vi "pitchVI.vi"() -> ()   [LabVIEW 2017]
uses:
  <vilib>/sound2/lvsound2.llb/Sound Output Task ID.ctl
  <vilib>/sound2/lvsound2.llb/Sound Output Write (DBL).vi
  <vilib>/sound2/lvsound2.llb/Sound File Write Open.vi
  <vilib>/sound2/lvsound2.llb/Sound File Write (DBL).vi
panel:
  in  "Clear":bool
  out "Sample Rate":dbl=48000.0
  in  "save":bool
  out "task ID out":T1=4294967295 format="%.0x"
  in  "Stop Play":bool
  in  "Pitch Shift \n(Octave)":i8
  in  "Shift":bool
  out "Right Channel":waveform(dbl)(graph)={"t0"=timestamp(0 s since 1904-01-01), "dt"=0.0020833333333333333, "Y"=[]}
  out "Left Channel":waveform(dbl)(graph)={"t0"=timestamp(0 s since 1904-01-01), "dt"=0.0020833333333333333, "Y"=[]}
  in  "waveform":dbl[][](array[numeric])
  in  "Stretch":bool
  in  "stop":bool
  in  "Play Signal":bool
  in  "Stretch Ratio":dbl=1.0
  in  "File to load":path
  # "Loneman's Phase Vocoder\nCopyright Jun D. Ouyang 06-06-2017"
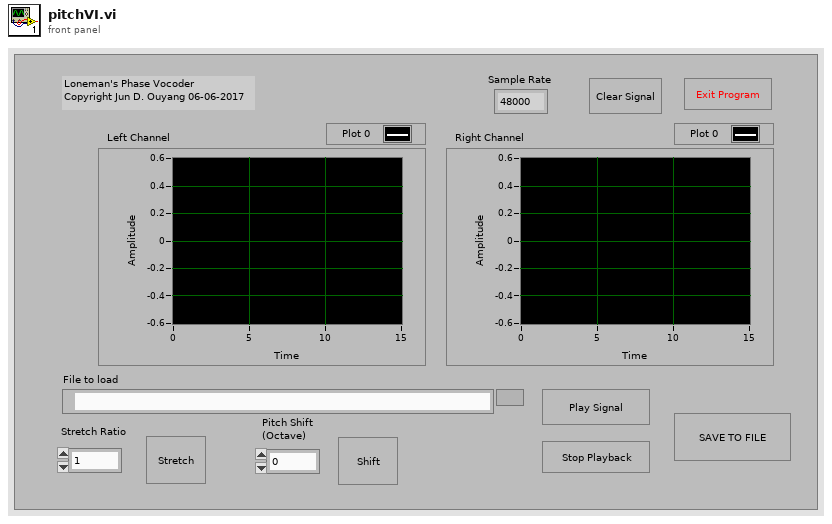
[diagram p1: front panel]
types:
  T1 = typedef "Sound Output Task ID.ctl" = u32
  T2 = typedef "Sound File Refnum.ctl" = refnum<file>
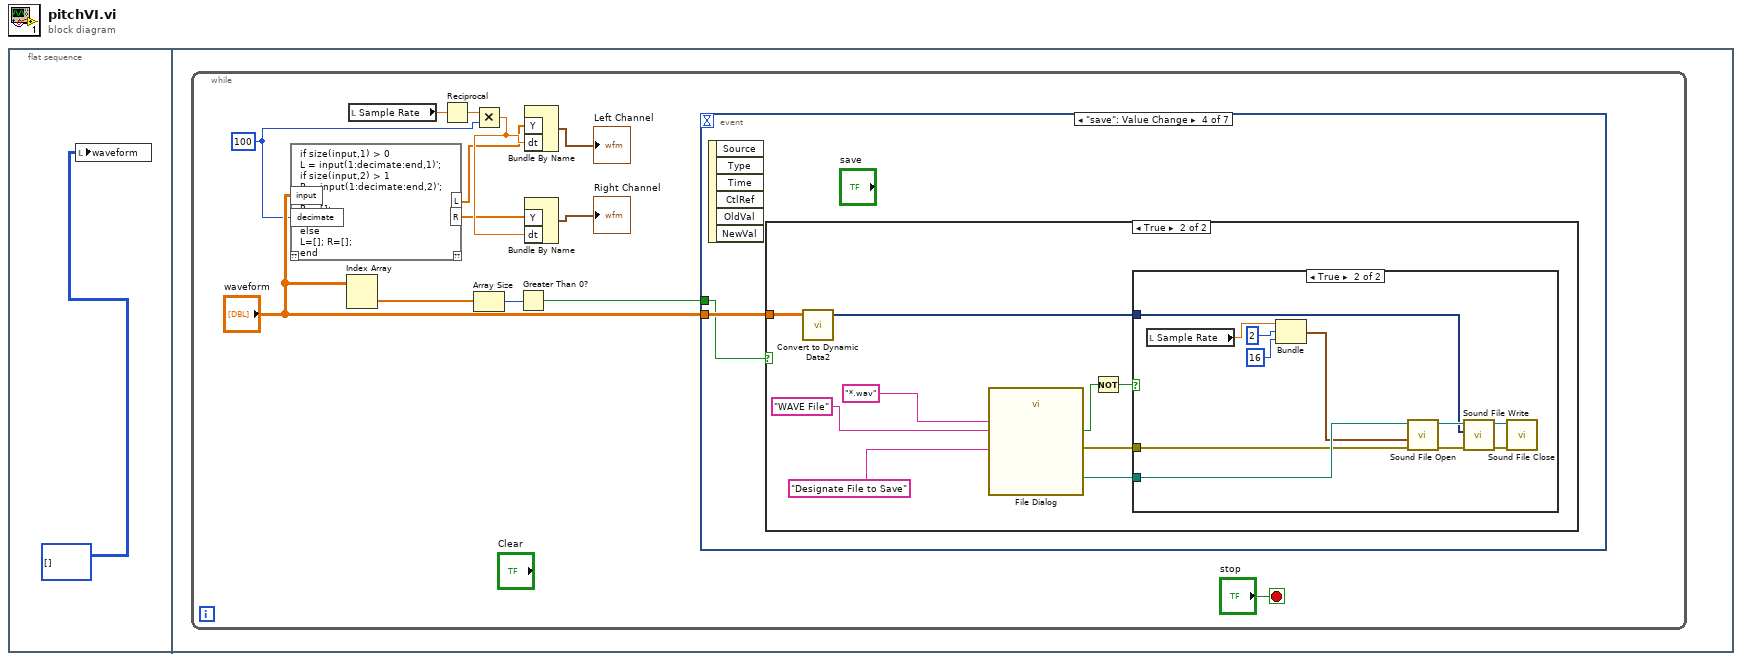
[diagram p0: block diagram]
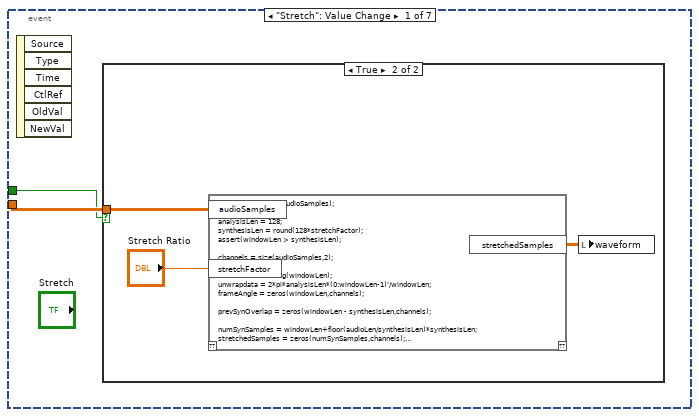
[diagram p2: hidden frame]
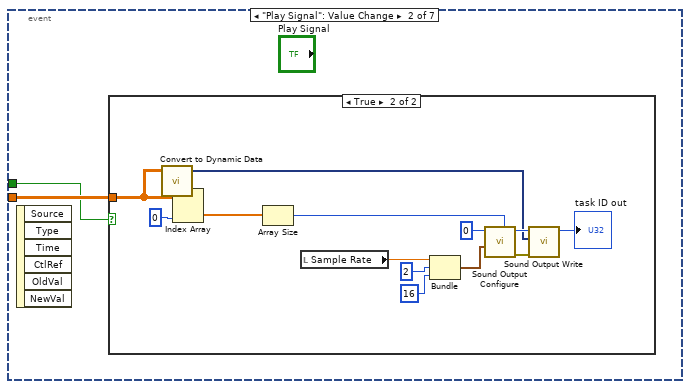
[diagram p4: hidden frame]
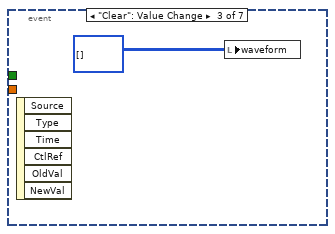
[diagram p6: hidden frame]
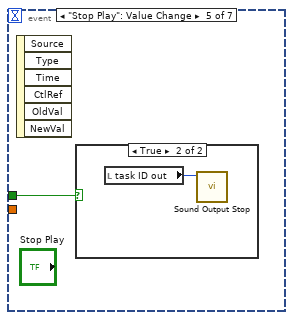
[diagram p9: hidden frame]
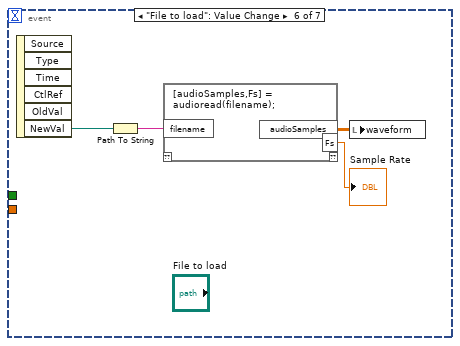
[diagram p11: hidden frame]
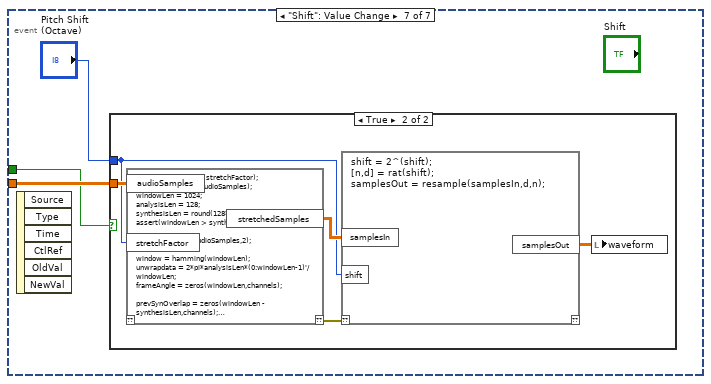
[diagram p12: hidden frame]
diagram:
  n1 = flat-sequence {
    frame #0 {
      n2 = local write "waveform"(i32[][] []) -> ()
    }
    frame #1 {
      n3 = while {
        stop <- "stop" stop-if-true
        w5 = 100
        n4 = script code="if size(input,1) > 0\nL = input(1:decimate:end,1)';\nif size(input,2) > 1\nR = input(1:decimate:end,2)';\nelse\nR = [];\nend\nelse\nL=[]; R=[];\nend"("input"="waveform", "decimate"=w5) -> ("L"=w3:dbl[], "R"=w2:dbl[])  [unwired: 1 in, 1 out]
        n5 = Index Array(array="waveform") -> (element=w14:dbl[])  [unwired: 2 in]
        n6 = local read "Sample Rate"() -> (w9:dbl)
        n7 = Reciprocal(x=w9) -> (1/x=w6:dbl)
        n8 = Multiply(x=w6, y=w5) -> (x*y=w4:dbl)
        n9 = Array Size(array=w14) -> (size(s)=w13:i32)
        n10 = Greater Than 0?(x=w13) -> (x > 0?=w10:bool)
        n11 = Bundle By Name("Y"=w3, "dt"=w4) -> (→"Left Channel":waveform(dbl))  [unwired: 1 in]
        n12 = Bundle By Name("Y"=w2, "dt"=w4) -> (→"Right Channel":waveform(dbl))  [unwired: 1 in]
        n13 = event shown="[3] \"save\": Value Change" {
          selector: _ -> [_ _ _ _ _ _ _]
          dyn-events: _ -> [_ _ _ _ _ _ _]
          timeout: _ -> [_ _ _ _ _ _ _]
          tunnel: "waveform" -> [w16 w21 _ w37 _ _ w66]
          tunnel: w10 -> [w15 w20 _ w36 w58 _ w64]
          event "Stretch": Value Change {
            n14 = event-data() -> ()  [unwired: 1 in, 6 out]
            n15 = case shown="True" w15 {
              tunnel: w16 -> [_ w18]
              frame False {
              }
              frame True {
                n16 = script code="audioLen = length(audioSamples);\nwindowLen = 1024;\nanalysisLen = 128;\nsynthesisLen = round(128*stretchFactor);\nassert(windowLen > synthesisLen);\n\nchannels = size(audioSamples,2);\n\nwindow = hamming(windowLen);\nunwrapdata = 2*pi*analysisLen*(0:windowLen-1)'/windowLen;\nframeAngle = zeros(windowLen,channels);\n\nprevSynOverlap = zeros(windowLen - synthesisLen,channels);\n\nnumSynSamples = windowLen+floor(audioLen/synthesisLen)*synthesisLen;\nstretchedSamples = zeros(numSynSamples,channels);\n\nindex = 1;\nsynIdex = 1;\nwhile index<audioLen\n    \n    prevFrameAngle = frameAngle;\n    \n    if index+windowLen < audioLen\n        frame = audioSamples(index:(index+windowLen-1),:);\n    else\n        frame = [audioSamples(index:end,:);zeros(windowLen+index-audioLen-1,channels)];\n    end\n    \n    frameTime = window.*frame;\n    frameFreq = fft(frameTime);\n    \n    frameAngle = angle(frameFreq);\n    frameMag = abs(frameFreq);\n    \n    frameAngleUnwrap = (frameAngle - prevFrameAngle) - unwrapdata;\n    frameAngleUnwrap = frameAngleUnwrap - round(frameAngleUnwrap/(2*pi))*2*pi;\n    frameAngleUnwrap = (frameAngleUnwrap + unwrapdata)*stretchFactor;\n    \n    if index == 1\n        synAngle = frameAngle;\n    else\n        synAngle = synAngle + frameAngleUnwrap;\n    end\n    \n    frameSynthFreq = frameMag.*exp(1j*synAngle);\n    frameSynthTime = real(ifft(frameSynthFreq)).*window;\n    \n    synOverlap = frameSynthTime(1:end-synthesisLen,:) + prevSynOverlap;\n    synFrame = [synOverlap;frameSynthTime(end-synthesisLen+1:end,:)];\n    \n    stretchedSamples(synIdex:synIdex+synthesisLen-1,:) = synFrame(1:synthesisLen,:);\n    prevSynOverlap = synFrame(synthesisLen+1:end,:);\n    index = index+analysisLen;\n    synIdex = synIdex+synthesisLen;\nend"("audioSamples"=w18, "stretchFactor"="Stretch Ratio") -> ("stretchedSamples"=w17:dbl[][])  [unwired: 1 in, 1 out]
                n17 = local write "waveform"(w17) -> ()
              }
            }
          }
          event "Play Signal": Value Change {
            n18 = event-data() -> ()  [unwired: 1 in, 6 out]
            n19 = case shown="True" w20 {
              tunnel: w21 -> [_ w26]
              frame False {
              }
              frame True {
                n20 = call "Convert to Dynamic Data"("2D Array"=w26) -> ("Dynamic Data Type"=w25:dynamicdata)  [unwired: 3 in]
                n21 = Index Array(array=w26, index (col)=0 ("disabled index (col)")) -> (element=w29:dbl[])  [unwired: 1 in]
                n22 = Array Size(array=w29) -> (size(s)=w28:i32)
                n23 = local read "Sample Rate"() -> (w22:dbl)
                n24 = Bundle("Sample Rate"=w22, 2, 16) -> (w31:cluster{"Sample Rate":dbl, i32, i32})  [unwired: 1 in]
                n25 = call <vilib>:"Sound Output Configure.vi"("number of samples/ch"=w28, "sound format"=w31, "device ID"=u32 0) -> ("error out"=w24:errorcluster, "task ID"=w27:T1)  [unwired: 7 in]
                n26 = call-poly <vilib>:"Sound Output Write.vi"("error in (no error)"=w24, "data"=w25, "task ID"=w27) -> ("task ID out"=→"task ID out":T1)  [unwired: 7 in, 1 out]
              }
            }
          }
          event "Clear": Value Change {
            n27 = event-data() -> ()  [unwired: 1 in, 6 out]
            n28 = local write "waveform"(i32[][] []) -> ()
          }
          event "save": Value Change {
            n29 = event-data() -> ()  [unwired: 1 in, 6 out]
            n30 = case shown="True" w36 {
              tunnel: w37 -> [_ w43]
              frame False {
              }
              frame True {
                n31 = call "Convert to Dynamic Data2"("2D Array"=w43) -> ("Dynamic Data Type"=w42:dynamicdata)  [unwired: 3 in]
                n32 = call "File Dialog"("prompt"="Designate File to Save", "pattern (all files)"="*.wav" ("pattern label"), "pattern label"="WAVE File" ("button label")) -> ("selected path"=w46:path, "cancelled"=w41:bool, "error out"=w45:errorcluster)  [unwired: 9 in, 1 out]
                n33 = Not(x=w41) -> (.not. x?=w40:bool)
                n34 = case shown="True" w40 {
                  tunnel: w46 -> [_ w57]
                  tunnel: w45 -> [_ w56]
                  tunnel: w42 -> [_ w51]
                  frame False {
                  }
                  frame True {
                    n35 = local read "Sample Rate"() -> (w48:dbl)
                    n36 = Bundle("Sample Rate"=w48, 2, 16) -> (w47:cluster{"Sample Rate":dbl, i32, i32})  [unwired: 1 in]
                    n37 = call-poly <vilib>:"Sound File Open.vi"("error in (no error)"=w56, "sound format"=w47, "path"=w57) -> ("error out"=w52:errorcluster, "sound file refnum"=w53:T2)  [unwired: 7 in]
                    n38 = call-poly <vilib>:"Sound File Write.vi"("error in (no error)"=w52, "data"=w51, "sound file refnum"=w53) -> ("error out"=w49:errorcluster, "sound file refnum out"=w50:T2)  [unwired: 7 in]
                    n39 = call <vilib>:"Sound File Close.vi"("error in (no error)"=w49, "sound file refnum"=w50) -> ()  [unwired: 9 in, 1 out]
                  }
                }
              }
            }
          }
          event "Stop Play": Value Change {
            n40 = event-data() -> ()  [unwired: 1 in, 6 out]
            n41 = case shown="True" w58 {
              frame False {
              }
              frame True {
                n42 = local read "task ID out"() -> (w59:T1)
                n43 = call <vilib>:"Sound Output Stop.vi"("task ID"=w59) -> ()  [unwired: 9 in, 2 out]
              }
            }
          }
          event "File to load": Value Change {
            n44 = event-data() -> ("NewVal"=w63:path)  [unwired: 1 in, 5 out]
            n45 = Path To String(path=w63) -> (string=w62:string)
            n46 = script code="[audioSamples,Fs] = audioread(filename);"("filename"=w62) -> ("audioSamples"=w61:dbl[][], "Fs"=→"Sample Rate":dbl)  [unwired: 1 in, 1 out]
            n47 = local write "waveform"(w61) -> ()
          }
          event "Shift": Value Change {
            n48 = event-data() -> ()  [unwired: 1 in, 6 out]
            n49 = case shown="True" w64 {
              tunnel: w66 -> [_ w70]
              tunnel: "Pitch Shift \n(Octave)" -> [_ w67]
              frame False {
              }
              frame True {
                n50 = script code="stretchFactor = 2^(stretchFactor);\naudioLen = length(audioSamples);\nwindowLen = 1024;\nanalysisLen = 128;\nsynthesisLen = round(128*stretchFactor);\nassert(windowLen > synthesisLen);\n\nchannels = size(audioSamples,2);\n\nwindow = hamming(windowLen);\nunwrapdata = 2*pi*analysisLen*(0:windowLen-1)'/windowLen;\nframeAngle = zeros(windowLen,channels);\n\nprevSynOverlap = zeros(windowLen - synthesisLen,channels);\n\nnumSynSamples = windowLen+floor(audioLen/synthesisLen)*synthesisLen;\nstretchedSamples = zeros(numSynSamples,channels);\n\nindex = 1;\nsynIdex = 1;\nwhile index<audioLen\n    \n    prevFrameAngle = frameAngle;\n    \n    if index+windowLen < audioLen\n        frame = audioSamples(index:(index+windowLen-1),:);\n    else\n        frame = [audioSamples(index:end,:);zeros(windowLen+index-audioLen-1,channels)];\n    end\n    \n    frameTime = window.*frame;\n    frameFreq = fft(frameTime);\n    \n    frameAngle = angle(frameFreq);\n    frameMag = abs(frameFreq);\n    \n    frameAngleUnwrap = (frameAngle - prevFrameAngle) - unwrapdata;\n    frameAngleUnwrap = frameAngleUnwrap - round(frameAngleUnwrap/(2*pi))*2*pi;\n    frameAngleUnwrap = (frameAngleUnwrap + unwrapdata)*stretchFactor;\n    \n    if index == 1\n        synAngle = frameAngle;\n    else\n        synAngle = synAngle + frameAngleUnwrap;\n    end\n    \n    frameSynthFreq = frameMag.*exp(1j*synAngle);\n    frameSynthTime = real(ifft(frameSynthFreq)).*window;\n    \n    synOverlap = frameSynthTime(1:end-synthesisLen,:) + prevSynOverlap;\n    synFrame = [synOverlap;frameSynthTime(end-synthesisLen+1:end,:)];\n    \n    stretchedSamples(synIdex:synIdex+synthesisLen-1,:) = synFrame(1:synthesisLen,:);\n    prevSynOverlap = synFrame(synthesisLen+1:end,:);\n    index = index+analysisLen;\n    synIdex = synIdex+synthesisLen;\nend"("audioSamples"=w70, "stretchFactor"=w67) -> ("??"=w68:errorcluster, "stretchedSamples"=w69:dbl[][])  [unwired: 1 in]
                n51 = script code="shift = 2^(shift);\n[n,d] = rat(shift);\nsamplesOut = resample(samplesIn,d,n);"("??"=w68, "samplesIn"=w69, "shift"=w67) -> ("samplesOut"=w71:dbl[][])  [unwired: 1 out]
                n52 = local write "waveform"(w71) -> ()
              }
            }
          }
        }
      }
    }
  }
